vi "AI Module.vi"(5 "acquire tag":T2, 7 "configuration tag":T3, 11 "exit tag":T2) -> (0 "done":bool=TRUE, 3 "wfm data stream":T1)   [LabVIEW 2019]
uses:
  <extravilib>/ChannelInstances/Tag-bool/))Channel.ctl
  <extravilib>/ChannelInstances/Tag-t'Measure and Log Settings.ctl'/))Channel.ctl
  subVIs/Measure and Log Settings.ctl
  subVIs/Simulated Signal Type.ctl
  <extravilib>/ChannelInstances/Stream-a[.](wfm(dbl))/)Channel.ctl
  <extravilib>/ChannelInstances/Tag-bool/Read With Abort.vi
  <extravilib>/ChannelInstances/Tag-t'Measure and Log Settings.ctl'/Read With Abort.vi
  <extravilib>/ChannelInstances/Stream-a[.](wfm(dbl))/Write With Abort.vi
  <extravilib>/ChannelInstances/Stream-a[.](wfm(dbl))/Endpoint.vi
  <extravilib>/ChannelInstances/Tag-bool/EndpointRead.vi
  <extravilib>/ChannelInstances/Tag-t'Measure and Log Settings.ctl'/EndpointRead.vi
  <extravilib>/ChannelInstances/Stream-a[.](wfm(dbl))/)Channel.vi
  <resource>/ChannelSupport/_ChannelSupport/WaitIfNeeded.vi
  <extravilib>/ChannelInstances/Tag-t'Measure and Log Settings.ctl'.lvlib
  <extravilib>/ChannelInstances/Stream-a[.](wfm(dbl)).lvlib
  <extravilib>/ChannelInstances/Tag-bool.lvlib
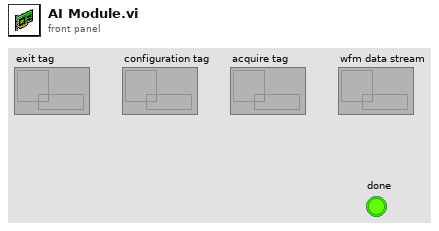
[diagram p1: front panel]
types:
  T1 = typedef "Stream-a[.](wfm(dbl)).lvlib/)Channel.ctl" = refnum<queue>
  T2 = typedef "Tag-bool.lvlib/))Channel.ctl" = refnum<queue>
  T3 = typedef "Tag-t'Measure and Log Settings.ctl'.lvlib/))Channel.ctl" = refnum<queue>
  T4 = typedef "Simulated Signal Type.ctl" = enum16{"Sine Wave", "Square Wave with Noise"}
  T5 = typedef "Measure and Log Settings.ctl" = cluster{"sample rate":dbl, "input range":dbl, "logfile path":path, "Simulated Signal":cluster{"signal type":T4, "frequency":dbl, "amplitude":dbl}}
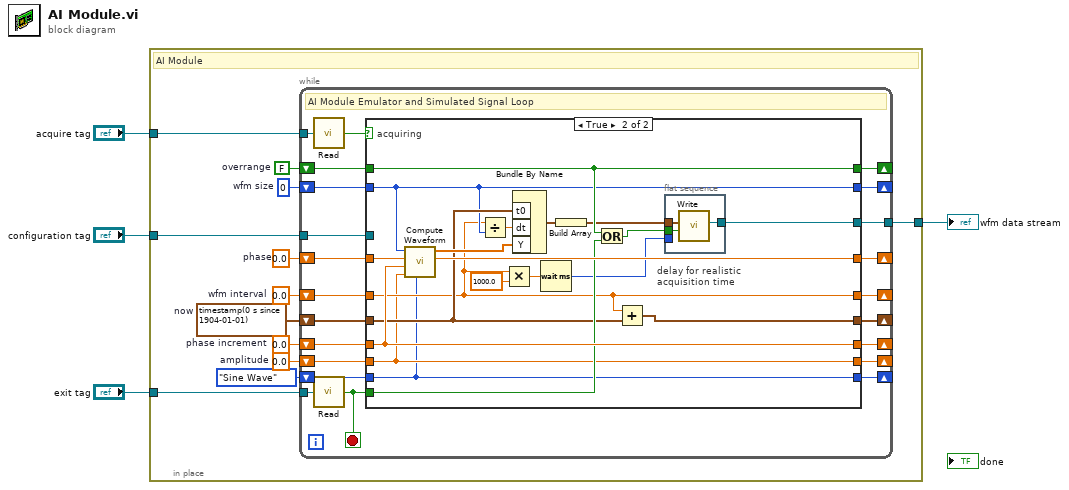
[diagram p0: block diagram]
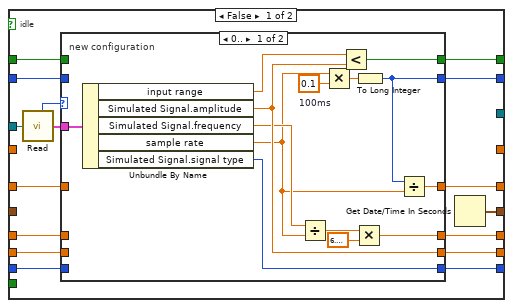
[diagram p2: hidden frame]
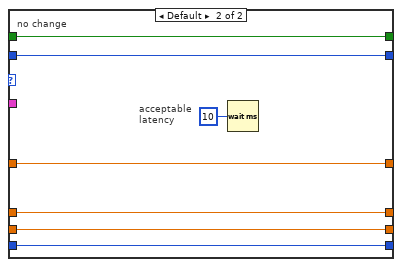
[diagram p3: hidden frame]
diagram:
  n1 = in-place {
    in-place-border: [w14] -> w1
    in-place-border: "acquire tag" -> [w13]
    in-place-border: "configuration tag" -> [w12]
    in-place-border: "exit tag" -> [w11]
    w6 = timestamp(0 s since 1904-01-01)  # now
    w7 = 0.0  # wfm interval
    w8 = 0  # wfm size
    w9 = FALSE  # overrange
    w10 = 0.0  # amplitude
    w16 = 0.0  # phase increment
    w15 = 0.0  # phase
    # "AI Module"
    n2 = while {
      shift-right: [w37] -> _
      shift-left: w15 -> [w38]
      tunnel: [w36] -> w14
      tunnel: w13 -> [w33]
      tunnel: w11 -> [w32]
      tunnel: w12 -> [w31]
      shift-right: [w30] -> _
      shift-left: w16 -> [w35]
      shift-right: [w29] -> _
      shift-left: Simulated_Signal_Type."Sine Wave" ("signal type") -> [w28]
      shift-right: [w27] -> _
      shift-left: w10 -> [w26]
      shift-right: [w25] -> _
      shift-left: w9 -> [w24]
      shift-right: [w23] -> _
      shift-left: w8 -> [w22]
      shift-right: [w21] -> _
      shift-left: w7 -> [w19]
      shift-right: [w20] -> _
      shift-left: w6 -> [w18]
      stop <- w17 stop-if-true
      # "AI Module Emulator and Simulated Signal Loop"
      n3 = call <extravilib>:"Read.vi"("channel"=w33) -> ("element"=w34:bool)  [unwired: 1 in, 1 out]
      n4 = call <extravilib>:"Read.vi"("channel"=w32) -> ("element"=w17:bool)  [unwired: 1 in, 1 out]
      n5 = case shown="True" w34 {
        tunnel: w38 -> [_ w95]
        tunnel: [_ w94] -> w37
        tunnel: [_ w83] -> w36
        tunnel: w35 -> [w54 w93]
        tunnel: w17 -> [_ w91]
        tunnel: w31 -> [w41 _]
        tunnel: [w53 w93] -> w30
        tunnel: [w52 w77] -> w29
        tunnel: w28 -> [w51 w77]
        tunnel: [w50 w78] -> w27
        tunnel: w26 -> [w49 w78]
        tunnel: [w48 w92] -> w25
        tunnel: w24 -> [w47 w92]
        tunnel: [w46 w86] -> w23
        tunnel: w22 -> [w45 w86]
        tunnel: [w44 w82] -> w21
        tunnel: [w43 w90] -> w20
        tunnel: w19 -> [w42 w82]
        tunnel: w18 -> [_ w88]
        frame False {
          # "idle"
          n6 = call <extravilib>:"Read.vi"("channel"=w41) -> ("missed"=w40:i32, "element"=w39:T5)  [unwired: 1 in]
          n7 = case shown="0.." w40 {
            tunnel: w39 -> [w68 _]
            tunnel: w54 -> [_ w75]
            tunnel: [w61 w75] -> w53
            tunnel: [w66 w74] -> w52
            tunnel: w51 -> [_ w74]
            tunnel: [w63 w73] -> w50
            tunnel: w49 -> [_ w73]
            tunnel: [w65 w72] -> w48
            tunnel: w47 -> [_ w72]
            tunnel: [w57 w71] -> w46
            tunnel: w45 -> [_ w71]
            tunnel: [w56 w70] -> w44
            tunnel: w42 -> [_ w70]
            frame 0.. {
              w60 = 0.1  # 100ms
              # "new configuration"
              n8 = Unbundle By Name(w68) -> ("input range"=w64:dbl, "Simulated Signal.amplitude"=w63:dbl, "Simulated Signal.frequency"=w58:dbl, "sample rate"=w55:dbl, "Simulated Signal.signal type"=w66:T4)
              n9 = Divide(x=w58, y=w55) -> (x/y=w62:dbl)
              n10 = Multiply(x=w55, y=w60) -> (x*y=w59:dbl)
              n11 = Less?(x=w64, y=w63) -> (x < y?=w65:bool)
              n12 = Multiply(x=w62, y=6.283185307179586) -> (x*y=w61:dbl)
              n13 = To Long Integer(number=w59) -> (32bit integer=w57:i32)
              n14 = Divide(x=w57, y=w55) -> (x/y=w56:dbl)
            }
            frame Default {
              # "acceptable\nlatency"
              # "no change"
              n15 = Wait (ms)(milliseconds to wait=u32 10) -> ()  [unwired: 1 out]
            }
          }
          n16 = Get Date/Time In Seconds() -> (seconds since 1Jan1904=w43:timestamp)
        }
        frame True {
          # "delay for realistic\nacquisition time"
          # "acquiring"
          n17 = call "Compute Waveform.vi"("signal type"=w77, "amplitude"=w78, "phase increment"=w93, "phase in"=w95, "wfm size"=w86) -> ("phase out"=w94:dbl, "wfm array"=w89:dbl[])  [unwired: 5 in]
          n18 = Divide(x=w82, y=w86) -> (x/y=w87:dbl)
          n19 = Multiply(x=w82, y=1000.0) -> (x*y=w80:dbl)
          n20 = Bundle By Name("t0"=w88, "dt"=w87, "Y"=w89) -> (w85:waveform(dbl))  [unwired: 1 in]
          n21 = Wait (ms)(milliseconds to wait=w80) -> (millisecond timer value=w76:u32)
          n22 = Build Array(w85) -> (w84:waveform(dbl)[])
          n23 = Or(x=w92, y=w91) -> (x .or. y?=w79:bool)
          n24 = Add(x=w82, y=w88) -> (x+y=w90:timestamp)
          n25 = flat-sequence {
            tunnel: w84 -> [w98]
            tunnel: [w97] -> w83
            tunnel: w79 -> [w96]
            tunnel: w76 -> [_]
            frame #0 {
              n26 = call <extravilib>:"Write.vi"("last element? (F)"=w96, "element"=w98) -> ("channel"=w97:T1)  [unwired: 7 in, 2 out]
            }
          }
        }
      }
    }
  }
  "wfm data stream" <- w1
